vi "Begin Mechanisms.vi"   [LabVIEW 2020]
uses:
  <vilib>/Rock Robotics/WPI/Solenoid/WPI_SolenoidChannel.ctl
  mechanisms.ctl
  <vilib>/Rock Robotics/WPI/ThirdParty/REV Robotics/REVLib/Typedef/Spark MAX Idle Mode.ctl
  <vilib>/Rock Robotics/WPI/ThirdParty/REV Robotics/REVLib/Typedef/Spark MAX Motor Type.ctl
  <vilib>/Rock Robotics/WPI/Solenoid/WPI_SolenoidOpenSingle.vi
  <vilib>/Rock Robotics/WPI/Utilities/WPI_GetSetVariantRefNum.vi
types:
  T1 = typedef "mechanisms.ctl" = string
  T2 = typedef "Spark MAX Idle Mode.ctl" = enum16{"Coast", "Brake"}
  T3 = typedef "Spark MAX Motor Type.ctl" = enum16{"Brushed", "Brushless"}
  T4 = typedef "WPI_SolenoidChannel.ctl" = enum8{"Solenoid 0", "Solenoid 1", "Solenoid 2", "Solenoid 3", "Solenoid 4", "Solenoid 5", "Solenoid 6", "Solenoid 7", "Solenoid 8", "Solenoid 9", "Solenoid 10", "Solenoid 11", "Solenoid 12", "Solenoid 13", "Solenoid 14", "Solenoid 15", "Invalid"}
  T5 = typedef "WPI_MotorControlDeviceRef.ctl" = cluster{"DeviceStatus":errorcluster, "Type":T6, "PWM":cluster{"PWM Channel":T7, "DeadBand":T8}, "CAN":cluster{"Device Number":u8, "SetOutput VI Ref":variant, "GetOutput VI Ref":variant, "Enable VI Ref":variant, "Disable VI Ref":variant, "Data":variant}, "Invert":bool, "DIO PWM":cluster{"PWM \"Enable\" Channel":T7, "DIOChannel":T9, "PWM Rate":dbl}}
  T6 = typedef "WPI_MotorControlType.ctl" = enum16{"PWM", "CAN", "DIO PWM"}
  T7 = typedef "FPGA_DIOPWMChannel.ctl" = enum8{"PWM 0", "PWM 1", "PWM 2", "PWM 3", "PWM 4", "PWM 5", "PWM 6", "PWM 7", "PWM 8", "PWM 9", "PWM MXP 0", "PWM MXP 1", "PWM MXP 2", "PWM MXP 3", "PWM MXP 4", "PWM MXP 5", "PWM MXP 6", "PWM MXP 7", "PWM MXP 8", "PWM MXP 9", "Invalid"}
  T8 = typedef "WPI_PWMDeadband.ctl" = cluster{"Name":string, "maxPositivePwm":i32, "minPositivePwm":i32, "centerPwm":i32, "maxNegativePwm":i32, "minNegativePwm":i32, "angularRange":u16}
  T9 = typedef "FPGA_DIOChannel.ctl" = enum8{"DIO 0", "DIO 1", "DIO 2", "DIO 3", "DIO 4", "DIO 5", "DIO 6", "DIO 7", "DIO 8", "DIO 9", "DIO MXP 0", "DIO MXP 1", "DIO MXP 2", "DIO MXP 3", "DIO MXP 4", "DIO MXP 5", "DIO MXP 6", "DIO MXP 7", "DIO MXP 8", "DIO MXP 9", "DIO MXP 10", "DIO MXP 11", "DIO MXP 12", "DIO MXP 13", "DIO MXP 14", "DIO MXP 15", "SPI Port CS1", "SPI Port CS2", "SPI Port CS3", "SPI Port MISO", "SPI Port MOSI", "Invalid"}
  T10 = typedef "WPI_SolenoidDevRef.ctl" = cluster{"DevStatus":errorcluster, "Pneumatics Control Module":u8, "Forward Solenoid Channel":T4, "Reverse Solenoid Channel":T4}
  T11 = typedef "WPI_CompressorDevRef.ctl" = cluster{"DevStatus":errorcluster, "Pneumatics Control Module":u8}
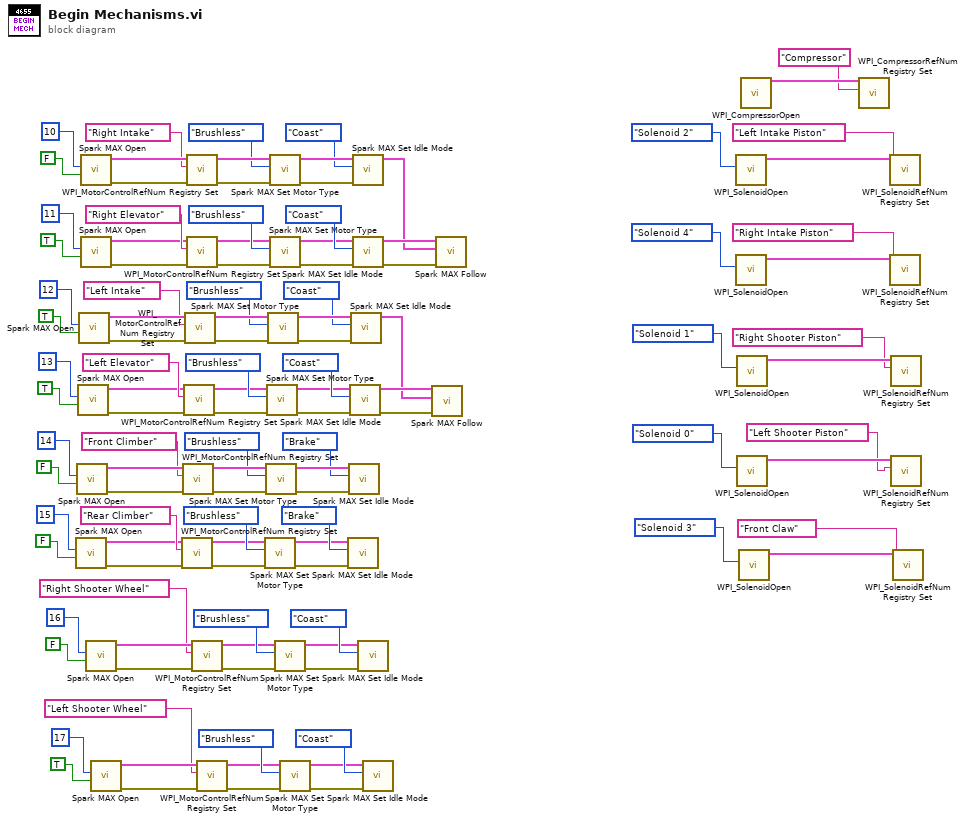
[diagram p0: block diagram]
diagram:
  n1 = call <vilib>:"Spark MAX Open.vi"("Invert"=FALSE, "Device Number"=u8 15) -> ("error out"=w47:errorcluster, "MotorControlDeviceRef"=w44:T5)  [unwired: 8 in]
  n2 = call <vilib>:"Spark MAX Open.vi"("Invert"=FALSE, "Device Number"=u8 14) -> ("error out"=w62:errorcluster, "MotorControlDeviceRef"=w65:T5)  [unwired: 8 in]
  n3 = call <vilib>:"Spark MAX Open.vi"("Invert"=TRUE, "Device Number"=u8 13) -> ("error out"=w69:errorcluster, "MotorControlDeviceRef"=w66:T5)  [unwired: 8 in]
  n4 = call <vilib>:"Spark MAX Open.vi"("Invert"=TRUE, "Device Number"=u8 12) -> ("error out"=w84:errorcluster, "MotorControlDeviceRef"=w87:T5)  [unwired: 8 in]
  n5 = call <vilib>:"Spark MAX Open.vi"("Invert"=FALSE, "Device Number"=u8 10) -> ("error out"=w108:errorcluster, "MotorControlDeviceRef"=w111:T5)  [unwired: 8 in]
  n6 = call <vilib>:"Spark MAX Open.vi"("Invert"=TRUE, "Device Number"=u8 11) -> ("error out"=w91:errorcluster, "MotorControlDeviceRef"=w88:T5)  [unwired: 8 in]
  n7 = call <vilib>:"Spark MAX Open.vi"("Invert"=FALSE, "Device Number"=u8 16) -> ("error out"=w16:errorcluster, "MotorControlDeviceRef"=w13:T5)  [unwired: 8 in]
  n8 = call <vilib>:"Spark MAX Open.vi"("Invert"=TRUE, "Device Number"=u8 17) -> ("error out"=w5:errorcluster, "MotorControlDeviceRef"=w2:T5)  [unwired: 8 in]
  n9 = call <vilib>:"WPI_MotorControlRefNum Registry Set.vi"("error in (no error)"=w47, "refnum name"=T1 "Rear Climber" ("Mechanism"), "MotorControlDevRef"=w44) -> ("error out"=w48:errorcluster, "MotorControlDevRef"=w45:T5)  [unwired: 7 in]
  n10 = call <vilib>:"WPI_MotorControlRefNum Registry Set.vi"("error in (no error)"=w62, "refnum name"=T1 "Front Climber" ("Mechanism"), "MotorControlDevRef"=w65) -> ("error out"=w61:errorcluster, "MotorControlDevRef"=w64:T5)  [unwired: 7 in]
  n11 = call <vilib>:"WPI_MotorControlRefNum Registry Set.vi"("error in (no error)"=w69, "refnum name"=T1 "Left Elevator" ("Mechanism"), "MotorControlDevRef"=w66) -> ("error out"=w70:errorcluster, "MotorControlDevRef"=w67:T5)  [unwired: 7 in]
  n12 = call <vilib>:"WPI_MotorControlRefNum Registry Set.vi"("error in (no error)"=w84, "refnum name"=T1 "Left Intake" ("Mechanism"), "MotorControlDevRef"=w87) -> ("error out"=w83:errorcluster, "MotorControlDevRef"=w86:T5)  [unwired: 7 in]
  n13 = call <vilib>:"WPI_MotorControlRefNum Registry Set.vi"("error in (no error)"=w108, "refnum name"=T1 "Right Intake" ("Mechanism"), "MotorControlDevRef"=w111) -> ("error out"=w107:errorcluster, "MotorControlDevRef"=w110:T5)  [unwired: 7 in]
  n14 = call <vilib>:"WPI_MotorControlRefNum Registry Set.vi"("error in (no error)"=w91, "refnum name"=T1 "Right Elevator" ("Mechanism"), "MotorControlDevRef"=w88) -> ("error out"=w92:errorcluster, "MotorControlDevRef"=w89:T5)  [unwired: 7 in]
  n15 = call <vilib>:"WPI_MotorControlRefNum Registry Set.vi"("error in (no error)"=w16, "refnum name"=T1 "Right Shooter Wheel" ("Mechanisms"), "MotorControlDevRef"=w13) -> ("error out"=w17:errorcluster, "MotorControlDevRef"=w14:T5)  [unwired: 7 in]
  n16 = call <vilib>:"WPI_MotorControlRefNum Registry Set.vi"("error in (no error)"=w5, "refnum name"=T1 "Left Shooter Wheel" ("Mechanisms"), "MotorControlDevRef"=w2) -> ("error out"=w6:errorcluster, "MotorControlDevRef"=w3:T5)  [unwired: 7 in]
  n17 = call <vilib>:"Spark MAX Set Motor Type.vi"("error in (no error)"=w48, "Motor Type"=Spark_MAX_Motor_Type."Brushless", "MotorControlDevRef"=w45) -> ("error out"=w49:errorcluster, "MotorControlDeviceRef"=w46:T5)  [unwired: 7 in]
  n18 = call <vilib>:"Spark MAX Set Motor Type.vi"("error in (no error)"=w61, "Motor Type"=Spark_MAX_Motor_Type."Brushless", "MotorControlDevRef"=w64) -> ("error out"=w60:errorcluster, "MotorControlDeviceRef"=w63:T5)  [unwired: 7 in]
  n19 = call <vilib>:"Spark MAX Set Motor Type.vi"("error in (no error)"=w70, "Motor Type"=Spark_MAX_Motor_Type."Brushless", "MotorControlDevRef"=w67) -> ("error out"=w71:errorcluster, "MotorControlDeviceRef"=w68:T5)  [unwired: 7 in]
  n20 = call <vilib>:"Spark MAX Set Motor Type.vi"("error in (no error)"=w83, "Motor Type"=Spark_MAX_Motor_Type."Brushless", "MotorControlDevRef"=w86) -> ("error out"=w82:errorcluster, "MotorControlDeviceRef"=w85:T5)  [unwired: 7 in]
  n21 = call <vilib>:"Spark MAX Set Motor Type.vi"("error in (no error)"=w107, "Motor Type"=Spark_MAX_Motor_Type."Brushless", "MotorControlDevRef"=w110) -> ("error out"=w106:errorcluster, "MotorControlDeviceRef"=w109:T5)  [unwired: 7 in]
  n22 = call <vilib>:"Spark MAX Set Motor Type.vi"("error in (no error)"=w92, "Motor Type"=Spark_MAX_Motor_Type."Brushless", "MotorControlDevRef"=w89) -> ("error out"=w93:errorcluster, "MotorControlDeviceRef"=w90:T5)  [unwired: 7 in]
  n23 = call <vilib>:"Spark MAX Set Motor Type.vi"("error in (no error)"=w17, "Motor Type"=Spark_MAX_Motor_Type."Brushless", "MotorControlDevRef"=w14) -> ("error out"=w18:errorcluster, "MotorControlDeviceRef"=w15:T5)  [unwired: 7 in]
  n24 = call <vilib>:"Spark MAX Set Motor Type.vi"("error in (no error)"=w6, "Motor Type"=Spark_MAX_Motor_Type."Brushless", "MotorControlDevRef"=w3) -> ("error out"=w7:errorcluster, "MotorControlDeviceRef"=w4:T5)  [unwired: 7 in]
  n25 = call <vilib>:"Spark MAX Set Idle Mode.vi"("error in (no error)"=w49, "Idle Mode"=Spark_MAX_Idle_Mode."Brake", "MotorControlDeviceRef in"=w46) -> ()  [unwired: 7 in, 2 out]
  n26 = call <vilib>:"Spark MAX Set Idle Mode.vi"("error in (no error)"=w60, "Idle Mode"=Spark_MAX_Idle_Mode."Brake", "MotorControlDeviceRef in"=w63) -> ()  [unwired: 7 in, 2 out]
  n27 = call <vilib>:"Spark MAX Set Idle Mode.vi"("error in (no error)"=w71, "Idle Mode"=Spark_MAX_Idle_Mode."Coast", "MotorControlDeviceRef in"=w68) -> ("error out"=w29:errorcluster, "MotorControlDeviceRef out"=w28:T5)  [unwired: 7 in]
  n28 = call <vilib>:"Spark MAX Set Idle Mode.vi"("error in (no error)"=w82, "Idle Mode"=Spark_MAX_Idle_Mode."Coast", "MotorControlDeviceRef in"=w85) -> ("MotorControlDeviceRef out"=w27:T5)  [unwired: 7 in, 1 out]
  n29 = call <vilib>:"Spark MAX Set Idle Mode.vi"("error in (no error)"=w106, "Idle Mode"=Spark_MAX_Idle_Mode."Coast", "MotorControlDeviceRef in"=w109) -> ("MotorControlDeviceRef out"=w30:T5)  [unwired: 7 in, 1 out]
  n30 = call <vilib>:"Spark MAX Set Idle Mode.vi"("error in (no error)"=w93, "Idle Mode"=Spark_MAX_Idle_Mode."Coast", "MotorControlDeviceRef in"=w90) -> ("error out"=w32:errorcluster, "MotorControlDeviceRef out"=w31:T5)  [unwired: 7 in]
  n31 = call <vilib>:"Spark MAX Set Idle Mode.vi"("error in (no error)"=w18, "Idle Mode"=Spark_MAX_Idle_Mode."Coast", "MotorControlDeviceRef in"=w15) -> ()  [unwired: 7 in, 2 out]
  n32 = call <vilib>:"Spark MAX Set Idle Mode.vi"("error in (no error)"=w7, "Idle Mode"=Spark_MAX_Idle_Mode."Coast", "MotorControlDeviceRef in"=w4) -> ()  [unwired: 7 in, 2 out]
  n33 = call <vilib>:"Spark MAX Follow.vi"("error in (no error)"=w29, "Master Controller"=w27, "MotorControlDeviceRef"=w28) -> ()  [unwired: 7 in, 2 out]
  n34 = call <vilib>:"Spark MAX Follow.vi"("error in (no error)"=w32, "Master Controller"=w30, "MotorControlDeviceRef"=w31) -> ()  [unwired: 7 in, 2 out]
  n35 = call-poly <vilib>:"WPI_SolenoidOpen.vi"("Solenoid Channel"=WPI_SolenoidChannel."Solenoid 2") -> ("SolenoidDevRef"=w100:T10)  [unwired: 9 in, 1 out]
  n36 = call-poly <vilib>:"WPI_SolenoidOpen.vi"("Solenoid Channel"=WPI_SolenoidChannel."Solenoid 4") -> ("SolenoidDevRef"=w41:T10)  [unwired: 9 in, 1 out]
  n37 = call-poly <vilib>:"WPI_SolenoidOpen.vi"("Solenoid Channel"=WPI_SolenoidChannel."Solenoid 1") -> ("SolenoidDevRef"=w38:T10)  [unwired: 9 in, 1 out]
  n38 = call-poly <vilib>:"WPI_SolenoidOpen.vi"("Solenoid Channel"=WPI_SolenoidChannel."Solenoid 0") -> ("SolenoidDevRef"=w37:T10)  [unwired: 9 in, 1 out]
  n39 = call-poly <vilib>:"WPI_SolenoidOpen.vi"("Solenoid Channel"=WPI_SolenoidChannel."Solenoid 3") -> ("SolenoidDevRef"=w34:T10)  [unwired: 9 in, 1 out]
  n40 = call <vilib>:"WPI_CompressorOpen.vi"() -> ("CompressorDevRef"=w24:T11)  [unwired: 14 in, 1 out]
  n41 = call <vilib>:"WPI_CompressorRefNum Registry Set.vi"("refnum name"="Compressor", "CompressorDevRef"=w24) -> ()  [unwired: 8 in, 2 out]
  n42 = call <vilib>:"WPI_SolenoidRefNum Registry Set.vi"("refnum name"=T1 "Left Intake Piston" ("Mechanism"), "SolenoidDevRef"=w100) -> ()  [unwired: 8 in, 2 out]
  n43 = call <vilib>:"WPI_SolenoidRefNum Registry Set.vi"("refnum name"=T1 "Right Intake Piston" ("Mechanism"), "SolenoidDevRef"=w41) -> ()  [unwired: 8 in, 2 out]
  n44 = call <vilib>:"WPI_SolenoidRefNum Registry Set.vi"("refnum name"=T1 "Right Shooter Piston" ("Mechanisms"), "SolenoidDevRef"=w38) -> ()  [unwired: 8 in, 2 out]
  n45 = call <vilib>:"WPI_SolenoidRefNum Registry Set.vi"("refnum name"=T1 "Left Shooter Piston" ("Mechanisms"), "SolenoidDevRef"=w37) -> ()  [unwired: 8 in, 2 out]
  n46 = call <vilib>:"WPI_SolenoidRefNum Registry Set.vi"("refnum name"=T1 "Front Claw" ("Mechanism"), "SolenoidDevRef"=w34) -> ()  [unwired: 8 in, 2 out]
